vi "VLC - Example (set pos).vi"() -> ()   [LabVIEW 2011]
uses:
  Program Files (x86)/VideoLAN/VLC/libvlc.dll
  System.Windows.Forms
panel:
  in  "PictureBox":refnum<k24>(container)
  in  "Goto":sgl
  in  "pause":bool
  out "Position":sgl
  out "Time (ms)":i32
  out "Ring":i32(ring) items=["IDLE/CLOSE", "OPENING", "BUFFERING", "PLAYING", "PAUSED", "STOPPING", "ENDED", "ERROR"]
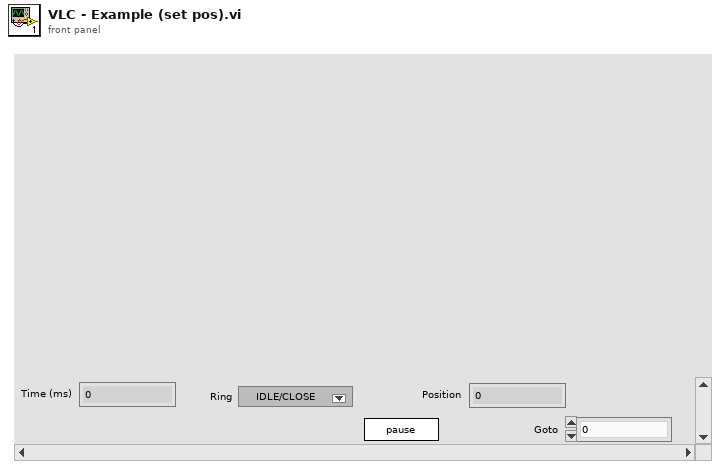
[diagram p1: front panel]
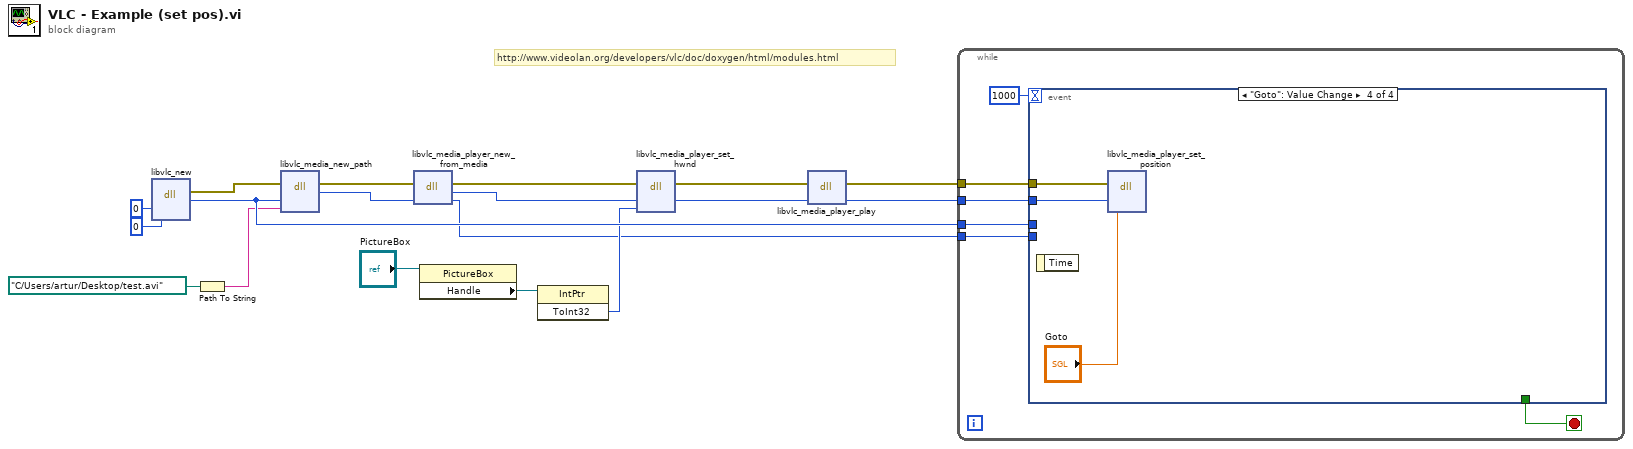
[diagram p0: block diagram]
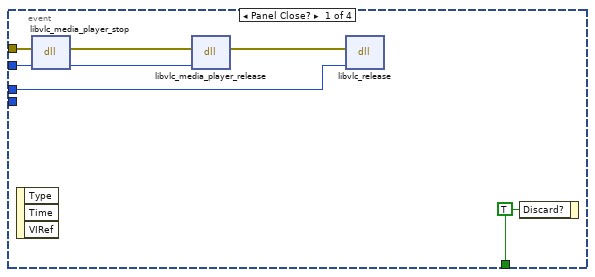
[diagram p2: hidden frame]
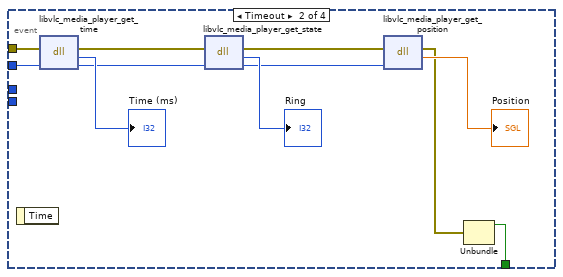
[diagram p3: hidden frame]
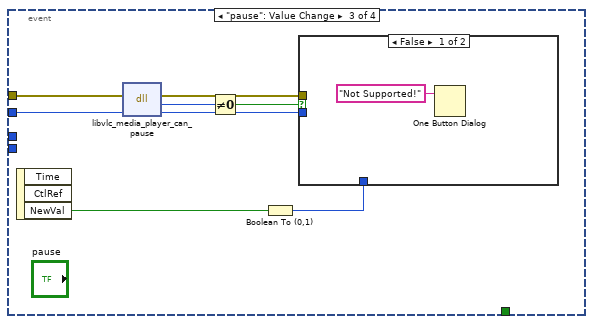
[diagram p4: hidden frame]
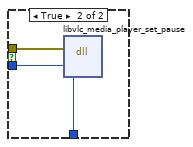
[diagram p5: hidden frame]
diagram:
  # "http://www.videolan.org/developers/vlc/doc/doxygen/html/modules.html"
  n1 = dll-call lib="C:/Program Files (x86)/VideoLAN/VLC/libvlc.dll" fn="libvlc_new"("argc"=0, "argv"=u8 0) -> (error out=w18:errorcluster, "return type"=w10:i32)  [unwired: 5 in, 1 out]
  n2 = Path To String(path=path "C:/Users/artur/Desktop/test.avi") -> (string=w5:string)
  n3 = dll-call lib="C:/Program Files (x86)/VideoLAN/VLC/libvlc.dll" fn="libvlc_media_new_path"(error in=w18, "p_instance"=w10, "path"=w5) -> (error out=w4:errorcluster, "return type"=w1:i32)  [unwired: 4 in, 1 out]
  n4 = dll-call lib="C:/Program Files (x86)/VideoLAN/VLC/libvlc.dll" fn="libvlc_media_player_new_from_media"(error in=w4, "p_md"=w1) -> (error out=w13:errorcluster, "return type"=w2:i32, "p_md"=w3:i32)  [unwired: 2 in, 1 out]
  n5 = property class="PictureBox"(reference="PictureBox") -> ("Handle"=w8:refnum<k24>)  [unwired: 1 in, 2 out]
  n6 = invoke class="IntPtr" method="ToInt32"(reference=w8) -> ("ToInt32"=w7:i32)  [unwired: 2 in, 2 out]
  n7 = dll-call lib="C:/Program Files (x86)/VideoLAN/VLC/libvlc.dll" fn="libvlc_media_player_set_hwnd"(error in=w13, "p_mi"=w2, "drawable"=w7) -> (error out=w16:errorcluster, "p_mi"=w17:i32)  [unwired: 4 in, 1 out]
  n8 = dll-call lib="C:/Program Files (x86)/VideoLAN/VLC/libvlc.dll" fn="libvlc_media_player_play"(error in=w16, "p_mi"=w17) -> (error out=w15:errorcluster, "p_mi"=w14:i32)  [unwired: 3 in, 1 out]
  n9 = while {
    tunnel: w15 -> [w24]
    tunnel: w14 -> [w23]
    tunnel: w3 -> [w20]
    tunnel: w10 -> [w19]
    stop <- w21 stop-if-true
    n10 = event shown="[3] \"Goto\": Value Change" {
      selector: _ -> [_ _ _ _]
      dyn-events: _ -> [_ _ _ _]
      timeout: 1000 -> [_ _ _ _]
      tunnel: w24 -> [w31 w42 w50 w57]
      tunnel: w23 -> [w30 w41 w49 w56]
      tunnel: w19 -> [w29 _ _ _]
      tunnel: [w27 w36 _ _] -> w21
      tunnel: w20 -> [_ _ _ _]
      event Panel Close? {
        w27 = TRUE ("Discard?")
        n11 = event-data() -> ()  [unwired: 1 in, 3 out]
        n12 = dll-call lib="C:/Program Files (x86)/VideoLAN/VLC/libvlc.dll" fn="libvlc_media_player_stop"(error in=w31, "p_mi"=w30) -> (error out=w26:errorcluster, "p_mi"=w25:i32)  [unwired: 3 in, 1 out]
        n13 = dll-call lib="C:/Program Files (x86)/VideoLAN/VLC/libvlc.dll" fn="libvlc_media_player_release"(error in=w26, "p_mi"=w25) -> (error out=w28:errorcluster)  [unwired: 4 in, 1 out]
        n14 = dll-call lib="C:/Program Files (x86)/VideoLAN/VLC/libvlc.dll" fn="libvlc_release"(error in=w28, "p_instnace"=w29) -> ()  [unwired: 4 in, 2 out]
        n15 = event-data("Discard?"=w27) -> ()  [unwired: 1 in, 1 out]
      }
      event Timeout {
        n16 = event-data() -> ()  [unwired: 1 in, 1 out]
        n17 = dll-call lib="C:/Program Files (x86)/VideoLAN/VLC/libvlc.dll" fn="libvlc_media_player_get_time"(error in=w42, "p_mi"=w41) -> (error out=w38:errorcluster, "return type"=→"Time (ms)":i32, "p_mi"=w37:i32)  [unwired: 2 in, 1 out]
        n18 = dll-call lib="C:/Program Files (x86)/VideoLAN/VLC/libvlc.dll" fn="libvlc_media_player_get_state"(error in=w38, "p_mi"=w37) -> (error out=w33:errorcluster, "return type"=→"Ring":i32, "p_mi"=w35:i32)  [unwired: 2 in, 1 out]
        n19 = dll-call lib="C:/Program Files (x86)/VideoLAN/VLC/libvlc.dll" fn="libvlc_media_player_get_position"(error in=w33, "p_mi"=w35) -> (error out=w32:errorcluster, "return type"=→"Position":sgl)  [unwired: 3 in, 1 out]
        n20 = Unbundle(w32) -> ("status"=w36:bool)  [unwired: 2 out]
      }
      event "pause": Value Change {
        n21 = event-data() -> ("NewVal"=w43:bool)  [unwired: 1 in, 2 out]
        n22 = dll-call lib="C:/Program Files (x86)/VideoLAN/VLC/libvlc.dll" fn="libvlc_media_player_can_pause" label="libvlc_media_player_set_pause"(error in=w50, "p_mi"=w49) -> (error out=w48:errorcluster, "return type"=w46:i32, "p_mi"=w47:i32)  [unwired: 2 in, 1 out]
        n23 = Not Equal To 0?(x=w46) -> (x != 0?=w45:bool)
        n24 = Boolean To (0,1)(Boolean=w43) -> (0, 1=w44:i16)
        n25 = case shown="False" w45 {
          tunnel: w48 -> [_ w54]
          tunnel: w47 -> [_ w53]
          tunnel: w44 -> [_ w52]
          frame False {
            n26 = One Button Dialog(message="Not Supported!") -> ()  [unwired: 1 in, 1 out]
          }
          frame True {
            n27 = dll-call lib="C:/Program Files (x86)/VideoLAN/VLC/libvlc.dll" fn="libvlc_media_player_set_pause"(error in=w54, "p_mi"=w53, "do_pause"=w52) -> ()  [unwired: 5 in, 2 out]
          }
        }
      }
      event "Goto": Value Change {
        n28 = event-data() -> ()  [unwired: 1 in, 1 out]
        n29 = dll-call lib="C:/Program Files (x86)/VideoLAN/VLC/libvlc.dll" fn="libvlc_media_player_set_position"(error in=w57, "p_mi"=w56, "f_pos"="Goto") -> ()  [unwired: 5 in, 2 out]
      }
    }
  }
